vi "Contour - Array Points to Contour.vi"(0 "Array Points":dbl[][](array[numeric])) -> (4 "Contour":T1)   [LabVIEW 2014]
doc: "Conversion from Array Points to Contour"
uses:
  MSC Image_class/controls/Contour.ctl
  MSC Image_class/MSC Image.lvclass
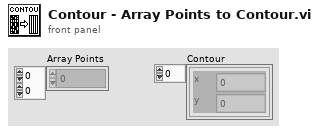
[diagram p1: front panel]
types:
  T1 = typedef "MSC Image.lvclass/Contour.ctl" = cluster{"x":i16, "y":i16}[]
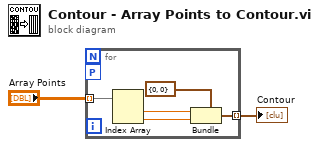
[diagram p0: block diagram]
diagram:
  n1 = for {
    tunnel: "Array Points" -> [w7] mode=indexing
    tunnel: [w4] -> w1 mode=indexing
    workers-P: _ -> [_]
    n2 = Index Array(array=w7) -> (element #1=w6:dbl, element #2=w5:dbl)  [unwired: 2 in]
    n3 = Bundle(cluster=cluster{"x":i16, "y":i16} {"x"=0, "y"=0} ("point"), "x"=w6, "y"=w5) -> (w4:cluster{"x":i16, "y":i16})
  }
  "Contour" <- w1
